vi "Close.vi"(8 "error in":errorcluster, 11 "Voltage Setpoint in":refnum<class "Voltage Setpoint.lvclass">) -> (0 "error out":errorcluster, 3 "Voltage Setpoint out":refnum<class "Voltage Setpoint.lvclass">)   [LabVIEW 2023, in "Voltage Setpoint.lvclass"]
uses:
  Voltage Setpoint.lvclass
  Parents/Setpoint/Setpoint.lvclass
  Voltage Setpoint.lvclass/Voltage Setpoint.ctl
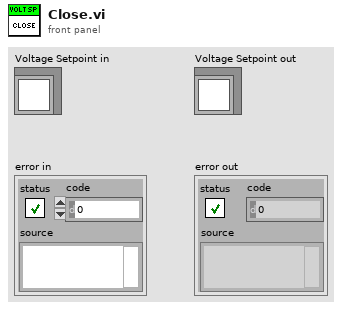
[diagram p1: front panel]
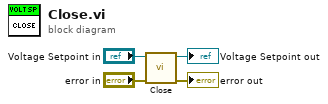
[diagram p0: block diagram]
diagram:
  n1 = call-parent "Close.vi"("error in"="error in", "Setpoint in"="Voltage Setpoint in") -> ("error out"=→"error out":errorcluster, "Setpoint out"=→"Voltage Setpoint out":refnum<class "Voltage Setpoint.lvclass">)  [unwired: 8 in]
